vi "Aerotech call forget acquire.vi"(8 "error in (no error)":errorcluster, 11 "AerotechStage in":refnum<class "AerotechStage.lvclass">) -> (0 "error out":errorcluster, 2 "Aerotech Acq Data":T1, 3 "AerotechStage out":refnum<class "AerotechStage.lvclass">)   [LabVIEW 2020, in "AerotechStage.lvclass"]
uses:
  AerotechStage.lvclass
  Aerotech Acq FGV Control.ctl
  Aerotech Acq FGV Function.ctl
  AerotechHardwareAcquire.vi
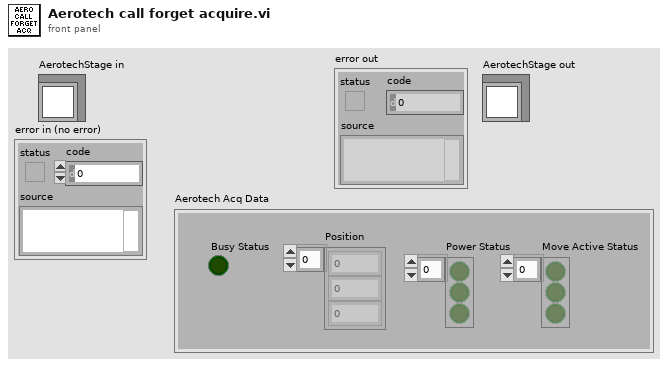
[diagram p1: front panel]
types:
  T1 = typedef "Aerotech Acq FGV Control.ctl" = cluster{"Position":dbl[], "Power Status":bool[], "Move Active Status":bool[], "Busy Status":bool}
  T2 = typedef "Aerotech Acq FGV Function.ctl" = enum16{"Clear", "Write", "Read"}
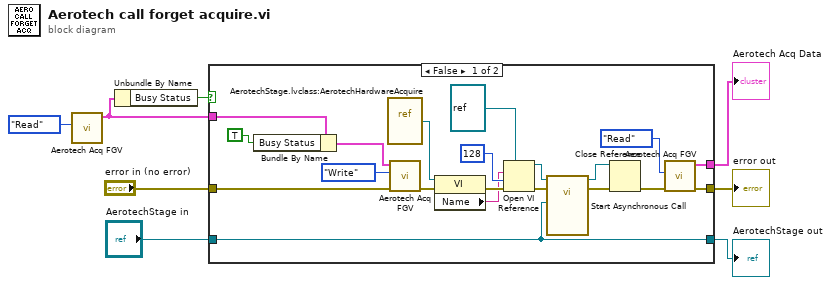
[diagram p0: block diagram]
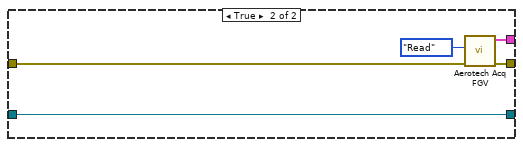
[diagram p2: hidden frame]
diagram:
  n1 = call "Aerotech Acq FGV.vi"("Function"=Aerotech_Acq_FGV_Function."Read") -> ("Aerotech Acq Data"=w4:T1)  [unwired: 9 in, 1 out]
  n2 = Unbundle By Name(w4) -> ("Busy Status"=w5:bool)
  n3 = case shown="False" w5 {
    tunnel: [w10 w33] -> w7
    tunnel: "AerotechStage in" -> [w10 w33]
    tunnel: w4 -> [w28 _]
    tunnel: "error in (no error)" -> [w24 w30]
    tunnel: [w11 w31] -> w2
    tunnel: [w9 w29] -> w1
    frame False {
      n4 = Bundle By Name(cluster=w28, "Busy Status"=TRUE) -> (w25:T1)
      n5 = vi-ref "AerotechStage.lvclass:AerotechHardwareAcquire.vi"() -> (w22:refnum<vi>)
      n6 = call "Aerotech Acq FGV.vi"("error in (no error)"=w24, "Function"=Aerotech_Acq_FGV_Function."Write", "Aerotech Acq Data"=w25) -> ("error out"=w23:errorcluster)  [unwired: 7 in, 1 out]
      n7 = property class="VI"(reference=w22, error in=w23) -> (error out=w20:errorcluster, "Name"=w14:string)  [unwired: 1 out]
      n8 = Open VI Reference(type specifier VI Refnum (for type only)=refnum<vi> refnum, vi path=w14, options=128, error in (no error)=w20) -> (vi reference=w17:refnum<vi>, error out=w19:errorcluster)  [unwired: 2 in]
      n9 = call-by-ref "Start Asynchronous Call"(reference=w17, error in=w19, "AerotechStage in"=w10) -> (reference out=w21:refnum<vi>, error out=w18:errorcluster)  [unwired: 9 in, 2 out]
      n10 = Close Reference(reference=w21, error in (no error)=w18) -> (error out=w12:errorcluster)
      n11 = call "Aerotech Acq FGV.vi"("error in (no error)"=w12, "Function"=Aerotech_Acq_FGV_Function."Read") -> ("error out"=w9:errorcluster, "Aerotech Acq Data"=w11:T1)  [unwired: 8 in]
    }
    frame True {
      n12 = call "Aerotech Acq FGV.vi"("error in (no error)"=w30, "Function"=Aerotech_Acq_FGV_Function."Read") -> ("error out"=w29:errorcluster, "Aerotech Acq Data"=w31:T1)  [unwired: 8 in]
    }
  }
  "AerotechStage out" <- w7
  "error out" <- w1
  "Aerotech Acq Data" <- w2
